vi "Check nonce.vi"(8 "error in (no error)":errorcluster, 10 "Challene data":T1, 11 "WampScramAuthenticator in":refnum<class "WampScramAuthenticator.lvclass">) -> (0 "error out":errorcluster, 2 "Challene data":T1, 3 "WampScramAuthenticator out":refnum<class "WampScramAuthenticator.lvclass">)   [LabVIEW 2020, in "wamplv.lvlib" / "WampScramAuthenticator.lvclass"]
uses:
  WampScramAuthenticator.lvclass
  TypeDefs/Challenge data.ctl
  WampScramAuthenticator.lvclass/WampScramAuthenticator.ctl
  <vilib>/Utility/error.llb/Error Cluster From Error Code.vi
  <vilib>/ErrorRing/Error Ring.xnode
  Utils/Utils.lvclass
  TypeDefs/HMAC parameters.ctl
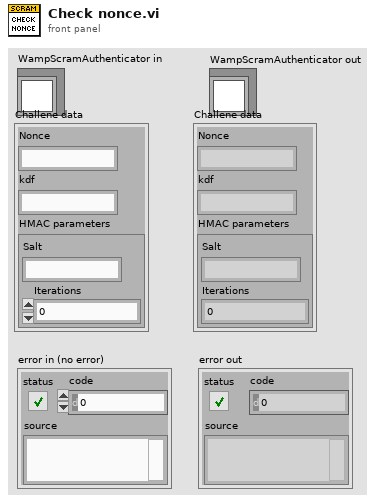
[diagram p1: front panel]
types:
  T1 = typedef "wamplv.lvlib/WampScramAuthenticator.lvclass/Challenge data.ctl" = cluster{"Nonce":string, "kdf":string, "HMAC parameters":T2}
  T2 = typedef "wamplv.lvlib/WampScramAuthenticator.lvclass/HMAC parameters.ctl" = cluster{"Salt":string, "Iterations":i32}
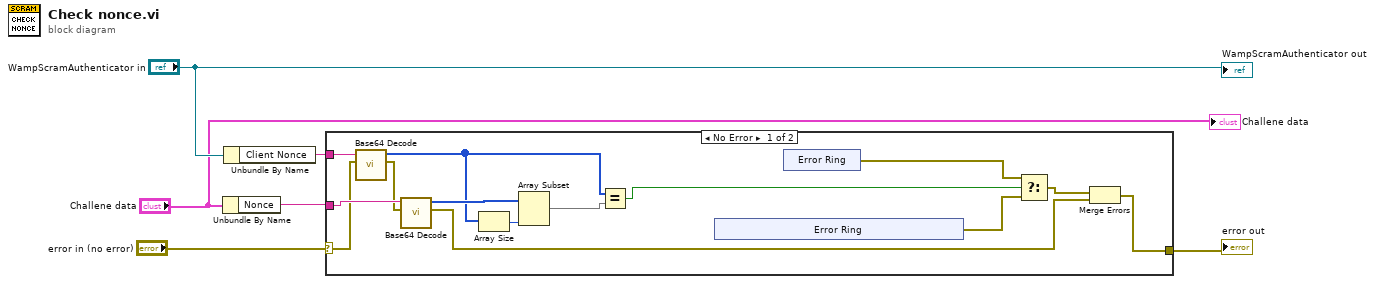
[diagram p0: block diagram]
diagram:
  n1 = Unbundle By Name("Challene data") -> ("Nonce"=w2:string)
  n2 = Unbundle By Name("WampScramAuthenticator in") -> ("Client Nonce"=w3:string)
  n3 = case shown="No Error" "error in (no error)" {
    selector: "error in (no error)" -> [w8 w26]
    tunnel: w2 -> [w15 _]
    tunnel: [w17 w26] -> w6
    tunnel: w3 -> [w16 _]
    frame No Error {
      n4 = call "Base64 Decode.vi"("error in (no error)"=w8, "string in (base64-encoded)"=w16) -> ("error out"=w7:errorcluster, "Byte array"=w12:u8[])  [unwired: 8 in]
      n5 = call "Base64 Decode.vi"("error in (no error)"=w7, "string in (base64-encoded)"=w15) -> ("error out"=w9:errorcluster, "Byte array"=w14:u8[])  [unwired: 8 in]
      n6 = Array Size(array=w12) -> (size(s)=w13:i32)
      n7 = Array Subset(array=w14, length=w13) -> (w11:u8[])  [unwired: 1 in]
      n8 = Equal?(x=w12, y=w11) -> (x = y?=w10:bool)
      n9 = xnode "Error Ring"() -> ("error out"=w19:errorcluster)
      n10 = xnode "Error Ring"() -> ("error out"=w20:errorcluster)
      n11 = Select(t=w20, s=w10, f=w19) -> (s? t:f=w18:errorcluster)
      n12 = Merge Errors(w18, w9) -> (w17:errorcluster)
    }
    frame Error {
    }
  }
  "error out" <- w6
  "WampScramAuthenticator out" <- "WampScramAuthenticator in"
  "Challene data" <- "Challene data"
